vi "IncrementalPCA.vi"(8 "error in":errorcluster) -> (0 "error out":errorcluster, 3 "out":refnum<class "IncrementalPCA.lvclass">)   [LabVIEW 2020]
doc: "Incremental principal components analysis (IPCA).\n\n Linear dimensionality reduction using Singular Value Decomposition of\n the data, keeping only the most significant singular vectors to\n project the data to a lower dimensional space. The input data is centered\n but not scaled for each feature before applying the SVD.\n\n Depending on the size of the input data, this algorithm can be much more\n memory efficient than a PCA, and allows sparse input.\n\n This algorithm has constant memory complexity, on the order\n of ``batch_size * n_features``, enabling use of np.memmap files without\n loading the entire file into memory. For sparse matrices, the input\n is converted to dense in batches (in order to be able to subtract the\n mean) which avoids storing the entire dense matrix at any one time.\n\n The computational overhead of each SVD is\n ``O(batch_size * n_features ** 2)``, but only 2 * batch_size samples\n remain in memory at a time. There will be ``n_samples / batch_size`` SVD\n computations to get the principal components, versus 1 large SVD of\n complexity ``O(n_samples * n_features ** 2)`` for PCA.\n\n Read more in the :ref:`User Guide <IncrementalPCA>`.\n\n .. versionadded:: 0.16\n\n Parameters\n ----------\n n_components : int, default=None\n Number of components to keep. If ``n_components`` is ``None``,\n then ``n_components`` is set to ``min(n_samples, n_features)``.\n\n whiten : bool, default=False\n When True (False by default) the ``components_`` vectors are divided\n by ``n_samples`` times ``components_`` to ensure uncorrelated outputs\n with unit component-wise variances.\n\n Whitening will remove some information from the transformed signal\n (the relative variance scales of the components) but can sometimes\n improve the predictive accuracy of the downstream estimators by\n making data respect some hard-wired assumptions.\n\n copy : bool, default=True\n If False, X will be overwritten. ``copy=False`` can be used to\n save memory but is unsafe for general use.\n\n batch_size : int, default=None\n The number of samples to use for each batch. Only used when calling\n ``fit``. If ``batch_size`` is ``None``, then ``batch_size``\n is inferred from the data and set to ``5 * n_features``, to provide a\n balance between approximation accuracy and memory consumption.\n\n Attributes\n ----------\n components_ : ndarray of shape (n_components, n_features)\n Components with maximum variance.\n\n explained_variance_ : ndarray of shape (n_components,)\n Variance explained by each of the selected components.\n\n explained_variance_ratio_ : ndarray of shape (n_components,)\n Percentage of variance explained by each of the selected components.\n If all components are stored, the sum of explained variances is equal\n to 1.0.\n\n singular_values_ : ndarray of shape (n_components,)\n The singular values corresponding to each of the selected components.\n The singular values are equal to the 2-norms of the ``n_components``\n variables in the lower-dimensional space.\n\n mean_ : ndarray of shape (n_features,)\n Per-feature empirical mean, aggregate over calls to ``partial_fit``.\n\n var_ : ndarray of shape (n_features,)\n Per-feature empirical variance, aggregate over calls to\n ``partial_fit``.\n\n noise_variance_ : float\n The estimated noise covariance following the Probabilistic PCA model\n from Tipping and Bishop 1999. See \"Pattern Recognition and\n Machine Learning\" by C. Bishop, 12.2.1 p. 574 or\n http://www.miketipping.com/papers/met-mppca.pdf.\n\n n_components_ : int\n The estimated number of components. Relevant when\n ``n_components=None``.\n\n n_samples_seen_ : int\n The number of samples processed by the estimator. Will be reset on\n new calls to fit, but increments across ``partial_fit`` calls.\n\n batch_size_ : int\n Inferred batch size from ``batch_size``.\n\n \nAvailable methods:\nFit\nFit Transform\nTransform\nGet Attributes\nGet Params\nSet Params"
uses:
  IncrementalPCA.lvclass
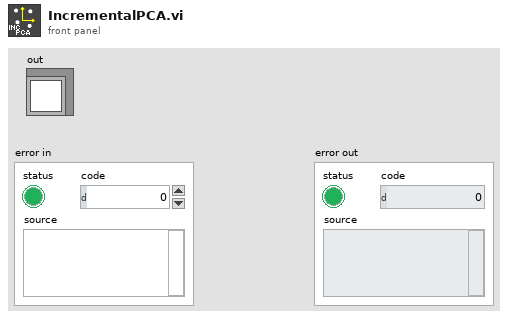
[diagram p1: front panel]
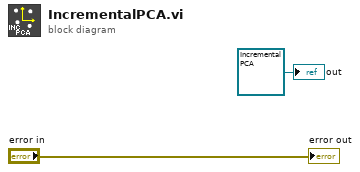
[diagram p0: block diagram]
diagram:
  "out" <- refnum<class "IncrementalPCA.lvclass"> refnum ("model")
  "error out" <- "error in"
